vi "Close-DOTNET.vi"(8 "error in (no error)":errorcluster, 11 "SM1000-control in":T1) -> (0 "error out":errorcluster, 1 "Succes?":bool, 3 "SM1000-control out":T1)   [LabVIEW 2013, in "SLMControl.lvlib" / "SM1000.lvclass"]
uses:
  SM1000.lvclass
  Object-reference.ctl
  SM1000.lvclass/SM1000.ctl
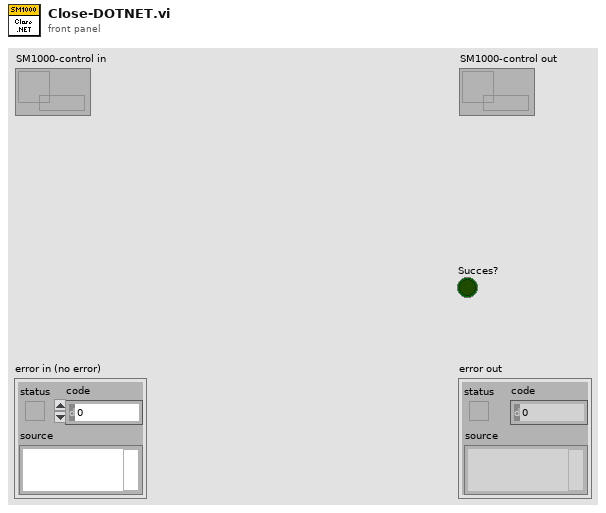
[diagram p1: front panel]
types:
  T1 = typedef "SLMControl.lvlib/SM1000.lvclass/Object-reference.ctl" = refnum<data-value>
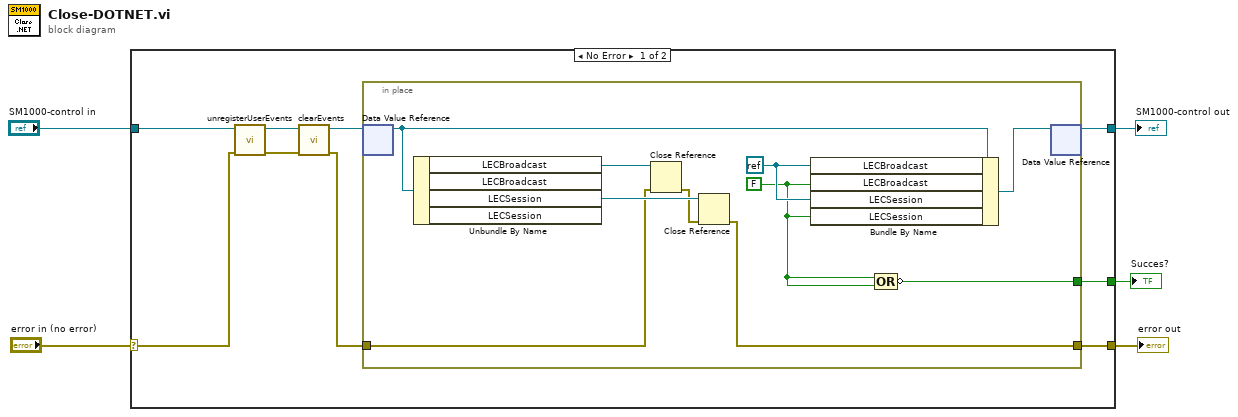
[diagram p0: block diagram]
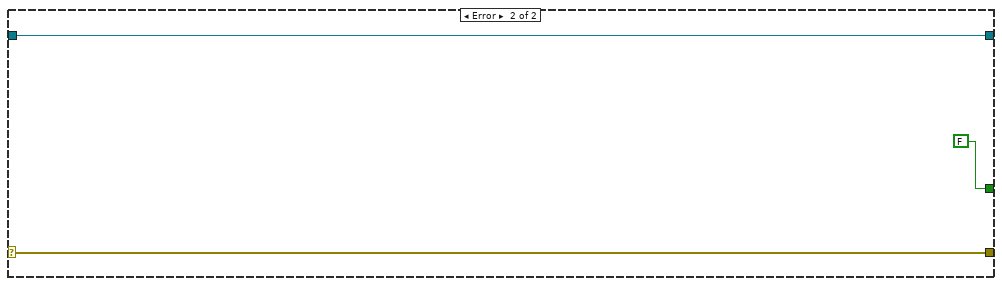
[diagram p2: hidden frame]
diagram:
  n1 = case shown="No Error" "error in (no error)" {
    selector: "error in (no error)" -> [w10 w27]
    tunnel: [w12 w27] -> w4
    tunnel: [w14 w26] -> w2
    tunnel: "SM1000-control in" -> [w11 w26]
    tunnel: [w13 FALSE] -> w1
    frame No Error {
      n2 = call "unregisterUserEvents.vi"("error in (no error)"=w10, "SM1000-control in"=w11) -> ("error out"=w7:errorcluster, "SM1000-control out"=w9:T1)  [unwired: 8 in]
      n3 = call "clearEvents.vi"("error in (no error)"=w7, "SM1000-control in"=w9) -> ("error out"=w6:errorcluster, "SM1000-control out"=w8:T1)  [unwired: 8 in]
      n4 = in-place {
        in-place-border: w6 -> [w17]
        in-place-border: [w23] -> w13
        in-place-border: [w15] -> w12
        w18 = FALSE
        w19 = refnum<k0> refnum
        n5 = in-place-dvr #1(w8) -> (w22:refnum<class "SM1000.lvclass">)  [unwired: 1 out]
        n6 = Unbundle By Name(w22) -> ("LECBroadcast"=w21:refnum<k24>, "LECSession"=w20:refnum<k24>)  [unwired: 2 out]
        n7 = Close Reference(reference=w21, error in (no error)=w17) -> (error out=w16:errorcluster)
        n8 = Close Reference(reference=w20, error in (no error)=w16) -> (error out=w15:errorcluster)
        n9 = Bundle By Name(cluster=w22, "LECBroadcast"=w19, "LECBroadcast"=w18, "LECSession"=w19, "LECSession"=w18) -> (w24:refnum<class "SM1000.lvclass">)
        n10 = Compound Arithmetic op=OR(w18, w18) -> (invert w23:bool)
        n11 = in-place-dvr #1(w24) -> (w14:T1)  [unwired: 1 out]
      }
    }
    frame Error {
    }
  }
  "error out" <- w4
  "SM1000-control out" <- w2
  "Succes?" <- w1
